vi "Main.vi"() -> ()   [LabVIEW 2021]
doc: "The myRIO Project template acquires acceleration data from the onboard accelerometer and displays the changes of acceleration values in a waveform chart."
uses:
  <vilib>/Instr/_visa.llb/VISA Configure Serial Port (Instr).vi
panel:
  in  "Stop Button":bool
  out "read buffer":string
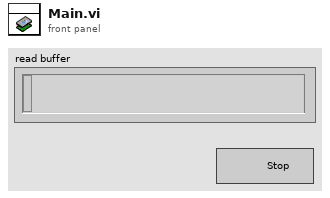
[diagram p1: front panel]
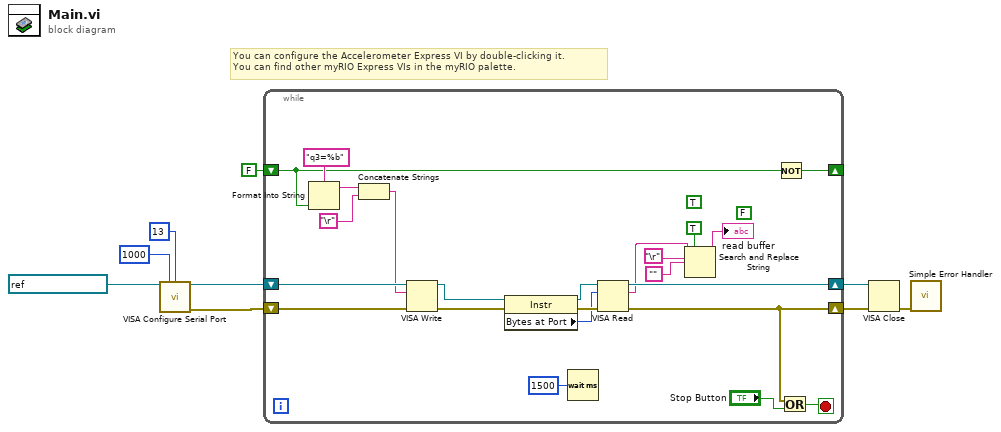
[diagram p0: block diagram]
diagram:
  # "You can configure the Accelerometer Express VI by double-clicking it.\nYou can find other myRIO Express VIs in the myRIO palette."
  n1 = call-poly "VISA Configure Serial Port"("VISA resource name"=refnum<visa-resource-name> "ASRL3::INSTR", "timeout (10sec)"=u32 1000, "termination char\n(0xA = '\\n' = LF)"=u8 13 ("termination char\n(0xA = '\\n' = LF)")) -> ("VISA resource name out"=w9:refnum<visa-resource-name>, "error out"=w8:errorcluster)  [unwired: 11 in]
  n2 = while {
    shift-right: [w27] -> w7
    shift-left: w9 -> [w32]
    shift-right: [w26] -> w6
    shift-left: w8 -> [w31]
    shift-right: [w15] -> _
    shift-left: FALSE -> [w13]
    stop <- w29 stop-if-true
    (unwired) FALSE ("replace all? (F)")
    (unwired) TRUE ("replace all? (F)")
    n3 = Format Into String(format string="q3=%b", w13) -> (resulting string=w12:string)  [unwired: 2 in, 1 out]
    n4 = Concatenate Strings(w12, "\r") -> (w10:string)
    n5 = VISA Write(VISA resource name=w32, write buffer=w10, error in (no error)=w31) -> (VISA resource name out=w16:refnum<visa-resource-name>, error out=w25:errorcluster)  [unwired: 1 out]
    n6 = property class="Instr"(reference=w16, error in=w25) -> (reference out=w20:refnum<visa-resource-name>, error out=w21:errorcluster, "Bytes at Port"=w19:u32)
    n7 = Wait (ms)(milliseconds to wait=u32 1500) -> ()  [unwired: 1 out]
    n8 = VISA Read(VISA resource name=w20, byte count=w19, error in (no error)=w21) -> (VISA resource name out=w27:refnum<visa-resource-name>, read buffer=w18:string, error out=w26:errorcluster)  [unwired: 1 out]
    n9 = Search and Replace String(replace all?=TRUE ("replace all? (F)"), input string=w18, search string="\r", replace string="") -> (result string=→"read buffer":string)  [unwired: 4 in, 3 out]
    n10 = Not(x=w13) -> (.not. x?=w15:bool)
    n11 = Or(x=w26, y="Stop Button") -> (x .or. y?=w29:bool)
  }
  n12 = VISA Close(VISA resource name=w7, error in (no error)=w6) -> (error out=w3:errorcluster)
  n13 = call <vilib>:"Simple Error Handler.vi"("error in (no error)"=w3) -> ()  [unwired: 4 in, 5 out]
